vi "ChirpSetupV2.vi"(8 "error in (no error)":errorcluster, 10 "R external(Ohm)":dbl=33.0, 11 "ChirpV2 in":refnum<class "ChirpV2.lvclass">) -> (0 "error out":errorcluster, 3 "ChirpV2 out":refnum<class "ChirpV2.lvclass">)   [LabVIEW 2014, in "ChirpV2.lvclass"]
uses:
  ChirpV2.lvclass
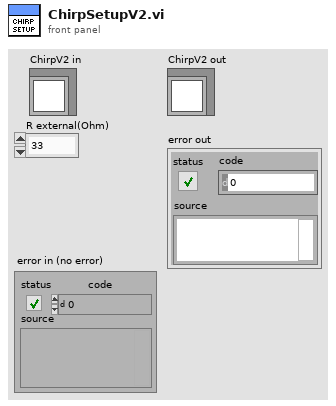
[diagram p1: front panel]
types:
  T1 = typedef "ChirpV2.lvclass/StateV2.ctl" = enum16{"WaitDC", "Initialization", "ChirpSetUp", "Wait", "ChirpMeasurement", "DFT", "WriteData", "Queue", "Ternimation"}
  T2 = cluster{"DC_Bias":dbl, "StartFreq":dbl, "Duration":dbl, "State":T1, "window ratio":dbl, "Final Freq":dbl}
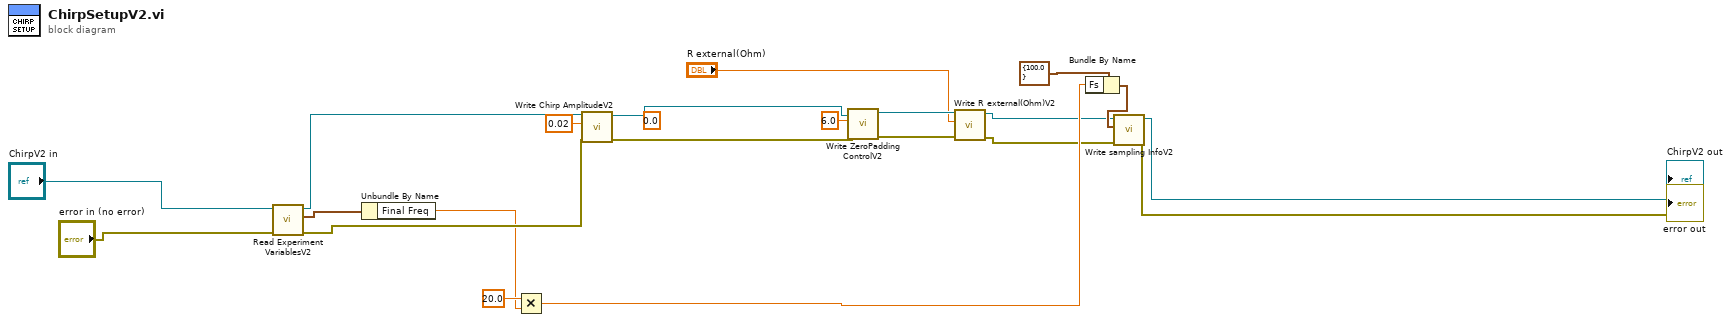
[diagram p0: block diagram]
diagram:
  (unwired) 0.0 ("DC_Bias")
  n1 = call-dynamic "Read Experiment VariablesV2.vi"("error in (no error)"="error in (no error)", "ChirpV2 in"="ChirpV2 in") -> ("error out"=w3:errorcluster, "Experiment Variables"=w4:T2, "ChirpV2 out"=w5:refnum<class "ChirpV2.lvclass">)  [unwired: 7 in]
  n2 = Unbundle By Name(w4) -> ("Final Freq"=w2:dbl)
  n3 = Multiply(x=20.0, y=w2) -> (x*y=w19:dbl)
  n4 = call-dynamic "Write Chirp AmplitudeV2.vi"("error in (no error)"=w3, "amplitude"=0.02, "ChirpV2 in"=w5) -> ("error out"=w8:errorcluster, "ChirpV2 out"=w9:refnum<class "ChirpV2.lvclass">)  [unwired: 7 in]
  n5 = call-dynamic "Write ZeroPadding ControlV2.vi"("error in (no error)"=w8, "ZeroPadding Control"=6.0, "ChirpV2 in"=w9) -> ("error out"=w13:errorcluster, "ChirpV2 out"=w10:refnum<class "ChirpV2.lvclass">)  [unwired: 7 in]
  n6 = call-dynamic "Write R external(Ohm)V2.vi"("error in (no error)"=w13, "R external(Ohm)"="R external(Ohm)", "ChirpV2 in"=w10) -> ("error out"=w15:errorcluster, "ChirpV2 out"=w14:refnum<class "ChirpV2.lvclass">)  [unwired: 7 in]
  n7 = Bundle By Name(cluster=cluster{"Fs":dbl} {"Fs"=100.0} ("sampling Info"), "Fs"=w19) -> (w18:cluster{"Fs":dbl})
  n8 = call-dynamic "Write sampling InfoV2.vi"("error in (no error)"=w15, "sampling Info"=w18, "ChirpV2 in"=w14) -> ("error out"=→"error out":errorcluster, "ChirpV2 out"=→"ChirpV2 out":refnum<class "ChirpV2.lvclass">)  [unwired: 7 in]
